vi "Heat1D_Form RHS.vi"(4 "Right BC":dbl, 6 "Left BC":dbl, 7 "step":i32, 8 "BC Type":i32, 9 "Coeff Array":dbl[](array[numeric]), 10 "F(x,t)":dbl[][](array[numeric]), 11 "U(n)":dbl[](array[numeric])) -> (3 "RHS":dbl[](array[numeric]))   [LabVIEW 2017, in "NI_PDE.lvlib"]
uses:
  <vilib>/gmath/NI_PDE.lvlib
  <vilib>/Analysis/2dsp.llb/1D Convolution (DBL).vi
  <vilib>/Analysis/NI_AALPro.lvlib
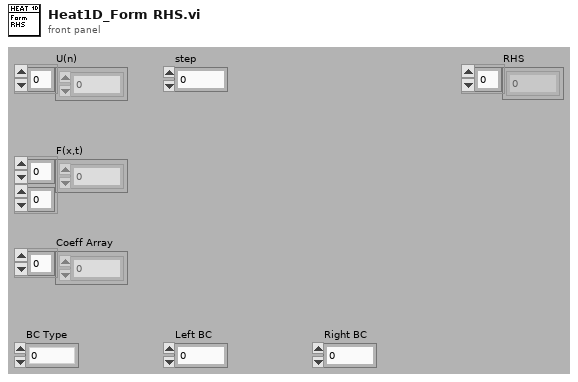
[diagram p1: front panel]
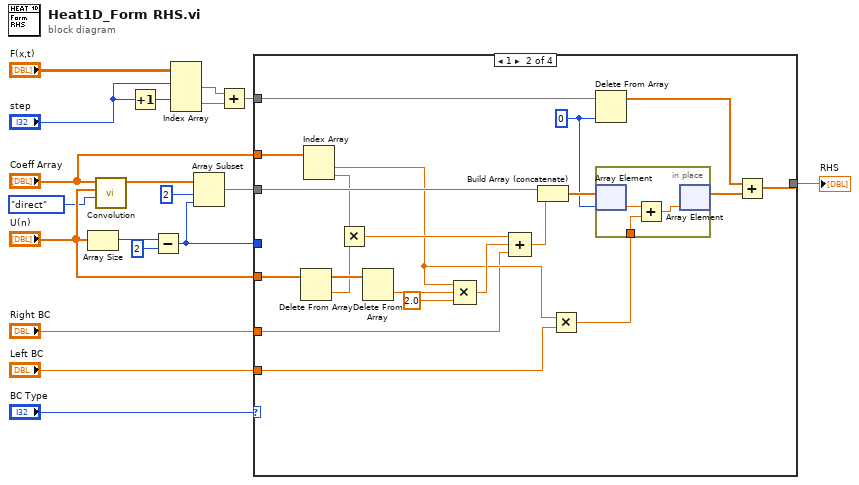
[diagram p0: block diagram]
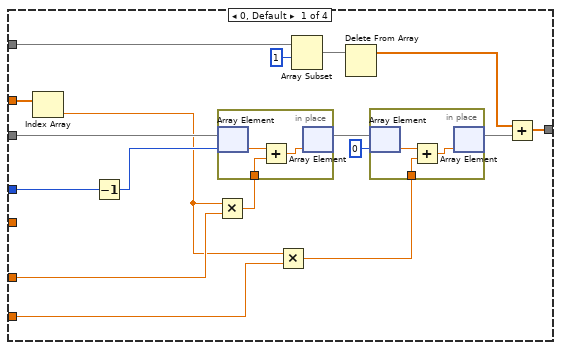
[diagram p2: hidden frame]
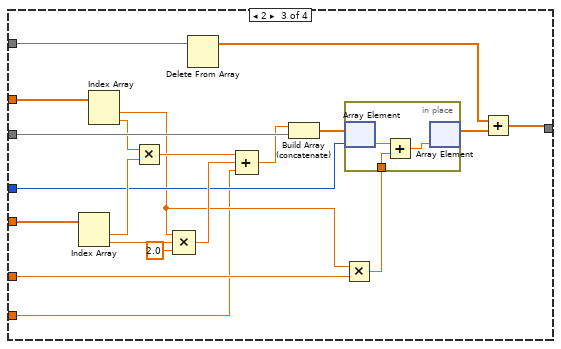
[diagram p3: hidden frame]
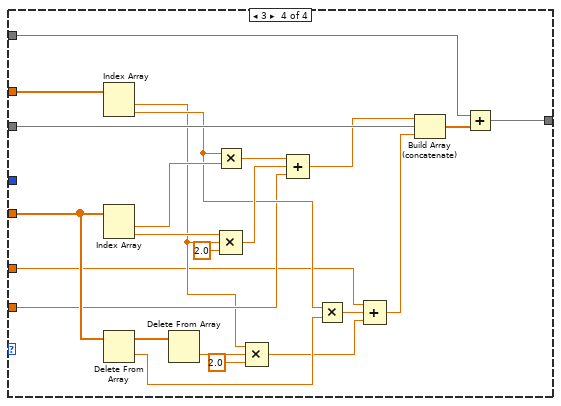
[diagram p4: hidden frame]
diagram:
  n1 = Array Size(array="U(n)") -> (size(s)=w11:i32)
  n2 = call-poly <vilib>:"Convolution.vi"("algorithm"=enum32{"direct", "frequency domain"}."direct", "Y"="U(n)", "X"="Coeff Array") -> ("X * Y"=w18:dbl[])  [unwired: 8 out]
  n3 = Increment(x="step") -> (x+1=w1:i32)
  n4 = Subtract(x=w11, y=2) -> (x-y=w13:i32)
  n5 = Index Array(array="F(x,t)", index (row) #1="step", index (row) #2=w1) -> (element #1=w6:dbl[], element #2=w5:dbl[])  [unwired: 2 in]
  n6 = Array Subset(array=w18, index=2, length=w13) -> (w10:dbl[])
  n7 = Add(x=w6, y=w5) -> (x+y=w3:dbl[])
  n8 = case shown="1" "BC Type" {
    tunnel: [w25 w45 w67 w96] -> w9
    tunnel: w10 -> [w31 w63 w83 w108]
    tunnel: w13 -> [w29 _ w74 _]
    tunnel: "Left BC" -> [w28 w53 w68 w97]
    tunnel: "Right BC" -> [w27 w46 w75 w90]
    tunnel: w3 -> [w24 w62 w80 w105]
    tunnel: "U(n)" -> [_ w61 w81 w104]
    tunnel: "Coeff Array" -> [w26 w50 w73 w100]
    frame 0, Default {
      n9 = Index Array(array=w26) -> (element=w22:dbl)  [unwired: 1 in]
      n10 = Decrement(x=w29) -> (x-1=w32:i32)
      n11 = Multiply(x=w22, y=w27) -> (x*y=w35:dbl)
      n12 = in-place {
        in-place-border: w35 -> [w42]
        n13 = in-place-array #1(w31, w32) -> (w41:dbl)
        n14 = Add(x=w41, y=w42) -> (x+y=w40:dbl)
        n15 = in-place-array #1(w40) -> (w33:dbl[])  [unwired: 1 out]
      }
      n16 = Multiply(x=w22, y=w28) -> (x*y=w36:dbl)
      n17 = Array Subset(array=w24, index=1) -> (w21:dbl[])  [unwired: 1 in]
      n18 = Delete From Array(array=w21) -> (array with subset deleted=w23:dbl[])  [unwired: 2 in, 1 out]
      n19 = in-place {
        in-place-border: w36 -> [w37]
        n20 = in-place-array #2(w33, 0) -> (w38:dbl)
        n21 = Add(x=w38, y=w37) -> (x+y=w39:dbl)
        n22 = in-place-array #2(w39) -> (w30:dbl[])  [unwired: 1 out]
      }
      n23 = Add(x=w23, y=w30) -> (x+y=w25:dbl[])
    }
    frame 1 {
      w44 = 0 ("index")
      n24 = Delete From Array(array=w61) -> (deleted portion=w57:dbl, array with subset deleted=w60:dbl[])  [unwired: 2 in]
      n25 = Index Array(array=w50) -> (element #1=w47:dbl, element #2=w49:dbl)  [unwired: 2 in]
      n26 = Multiply(x=w49, y=w57) -> (x*y=w58:dbl)
      n27 = Delete From Array(array=w60) -> (deleted portion=w48:dbl)  [unwired: 2 in, 1 out]
      n28 = Compound Arithmetic op=MULTIPLY(w47, w48, 2.0 ("value")) -> (w59:dbl)
      n29 = Compound Arithmetic op=ADD(w58, w59, w46) -> (w56:dbl)
      n30 = Build Array (concatenate)(w63, w56) -> (w55:dbl[])
      n31 = Multiply(x=w47, y=w53) -> (x*y=w51:dbl)
      n32 = Delete From Array(array=w62, index=w44) -> (array with subset deleted=w43:dbl[])  [unwired: 1 in, 1 out]
      n33 = in-place {
        in-place-border: w51 -> [w64]
        n34 = in-place-array #3(w55, w44) -> (w65:dbl)
        n35 = Add(x=w65, y=w64) -> (x+y=w66:dbl)
        n36 = in-place-array #3(w66) -> (w54:dbl[])  [unwired: 1 out]
      }
      n37 = Add(x=w43, y=w54) -> (x+y=w45:dbl[])
    }
    frame 2 {
      n38 = Index Array(array=w81) -> (element #1=w86:dbl, element #2=w71:dbl)  [unwired: 2 in]
      n39 = Index Array(array=w73) -> (element #1=w70:dbl, element #2=w72:dbl)  [unwired: 2 in]
      n40 = Multiply(x=w72, y=w86) -> (x*y=w85:dbl)
      n41 = Compound Arithmetic op=MULTIPLY(w70, w71, 2.0 ("value")) -> (w84:dbl)
      n42 = Delete From Array(array=w80) -> (array with subset deleted=w79:dbl[])  [unwired: 2 in, 1 out]
      n43 = Compound Arithmetic op=ADD(w85, w84, w68) -> (w82:dbl)
      n44 = Build Array (concatenate)(w82, w83) -> (w77:dbl[])
      n45 = Multiply(x=w70, y=w75) -> (x*y=w78:dbl)
      n46 = in-place {
        in-place-border: w78 -> [w89]
        n47 = in-place-array #4(w77, w74) -> (w88:dbl)
        n48 = Add(x=w88, y=w89) -> (x+y=w87:dbl)
        n49 = in-place-array #4(w87) -> (w76:dbl[])  [unwired: 1 out]
      }
      n50 = Add(x=w79, y=w76) -> (x+y=w67:dbl[])
    }
    frame 3 {
      n51 = Index Array(array=w100) -> (element #1=w92:dbl, element #2=w99:dbl)  [unwired: 2 in]
      n52 = Index Array(array=w104) -> (element #1=w112:dbl, element #2=w111:dbl)  [unwired: 2 in]
      n53 = Delete From Array(array=w104) -> (deleted portion=w95:dbl, array with subset deleted=w103:dbl[])  [unwired: 2 in]
      n54 = Delete From Array(array=w103) -> (deleted portion=w94:dbl)  [unwired: 2 in, 1 out]
      n55 = Multiply(x=w99, y=w112) -> (x*y=w110:dbl)
      n56 = Compound Arithmetic op=MULTIPLY(w111, w92, 2.0 ("value")) -> (w109:dbl)
      n57 = Compound Arithmetic op=MULTIPLY(w92, w94, 2.0 ("value")) -> (w91:dbl)
      n58 = Compound Arithmetic op=ADD(w110, w109, w97) -> (w107:dbl)
      n59 = Multiply(x=w99, y=w95) -> (x*y=w102:dbl)
      n60 = Compound Arithmetic op=ADD(w90, w102, w91) -> (w101:dbl)
      n61 = Build Array (concatenate)(w107, w108, w101) -> (w106:dbl[])
      n62 = Add(x=w105, y=w106) -> (x+y=w96:dbl[])
    }
  }
  "RHS" <- w9
